vi "Configure Multi Eval Meas Limit SEM OBW.vi"(7 "Limit OBW (40e+6)":dbl=40000000.0 format="%^.3e", 8 "error in (no error)":errorcluster, 9 "Limit OBW Enabled (Value)":i32(ring)=2 items=["Off", "On", "Value"], 10 "Instance (1)":T1=1, 11 "VISA resource name":refnum<visa-resource-name>) -> (0 "error out":errorcluster, 3 "VISA resource name out":refnum<visa-resource-name>)   [LabVIEW 2020, in "Rohde&Schwarz CMWXP NR FR1 Measurement.lvlib"]
doc: "Defines an upper limit for the occupied bandwidth, for EN-DC measurements.\n\nAttributes:\nRSCMWXPNRFR1M_ATTR_MULTI_EVAL_MEAS_LIMIT_SEM_OBW_ENABLED\nRSCMWXPNRFR1M_ATTR_MULTI_EVAL_MEAS_LIMIT_SEM_OBW\n\nRemote-control command:\nCONFigure:NRSub:MEAS<i>:MEValuation:LIMit:SEMask:OBWLimit:ENDC"
uses:
  <instrlib>/Rohde&Schwarz CMWXP NR FR1 Measurement/Rohde&Schwarz CMWXP NR FR1 Measurement.lvlib
  <instrlib>/Rohde&Schwarz CMWXP NR FR1 Measurement/Private/_Instance.ctl
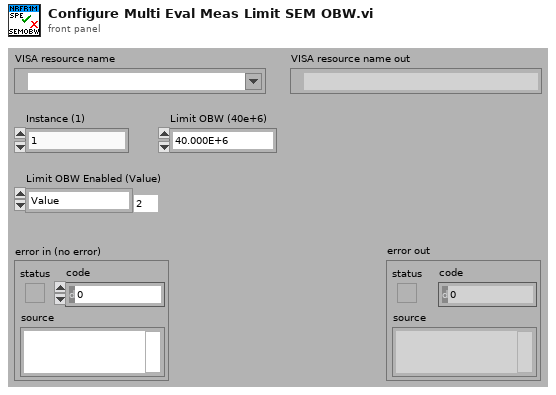
[diagram p1: front panel]
types:
  T1 = typedef "Rohde&Schwarz CMWXP NR FR1 Measurement.lvlib/_Instance.ctl" = i32
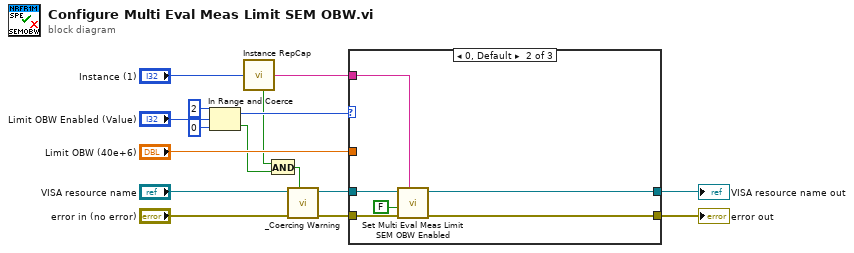
[diagram p0: block diagram]
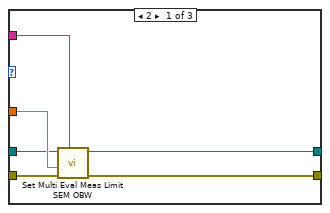
[diagram p2: hidden frame]
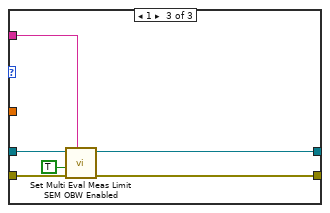
[diagram p3: hidden frame]
diagram:
  n1 = In Range and Coerce(upper limit=2, x="Limit OBW Enabled (Value)", lower limit=0) -> (coerced(x)=w12:i32, In Range?=w1:bool)
  n2 = call <instrlib>:"Instance RepCap.vi"("Instance In"="Instance (1)") -> ("In Range?"=w2:bool, "RepCap Identifier Out"=w8:string)  [unwired: 1 in]
  n3 = And(x=w2, y=w1) -> (x .and. y?=w3:bool)
  n4 = call <instrlib>:"_Coercing Warning.vi"("In Range?"=w3, "error in (no error)"="error in (no error)", "VISA resource name"="VISA resource name") -> ("error out"=w16:errorcluster, "VISA resource name out"=w15:refnum<visa-resource-name>)  [unwired: 7 in]
  n5 = case shown="0, Default" w12 {
    tunnel: [w22 w28 w34] -> w4
    tunnel: [w21 w27 w33] -> w5
    tunnel: "Limit OBW (40e+6)" -> [w20 _ _]
    tunnel: w16 -> [w19 w26 w32]
    tunnel: w15 -> [w18 w25 w31]
    tunnel: w8 -> [w17 w24 w30]
    frame 2 {
      n6 = call "Set Multi Eval Meas Limit SEM OBW"("Repeated Capabilities"=w17, "error in (no error)"=w19, "Multi Eval Meas Limit SEM OBW (0.0)"=w20, "instrument handle"=w18) -> ("error out"=w22:errorcluster, "instrument handle out"=w21:refnum<visa-resource-name>)  [unwired: 6 in]
    }
    frame 0, Default {
      n7 = call "Set Multi Eval Meas Limit SEM OBW Enabled"("Repeated Capabilities"=w24, "error in (no error)"=w26, "Multi Eval Meas Limit SEM OBW Enabled (OFF)"=FALSE ("Multi Eval Meas Limit OBW Enabled (OFF)"), "instrument handle"=w25) -> ("error out"=w28:errorcluster, "instrument handle out"=w27:refnum<visa-resource-name>)  [unwired: 6 in]
    }
    frame 1 {
      n8 = call "Set Multi Eval Meas Limit SEM OBW Enabled"("Repeated Capabilities"=w30, "error in (no error)"=w32, "Multi Eval Meas Limit SEM OBW Enabled (OFF)"=TRUE ("Multi Eval Meas Limit OBW Enabled (OFF)"), "instrument handle"=w31) -> ("error out"=w34:errorcluster, "instrument handle out"=w33:refnum<visa-resource-name>)  [unwired: 6 in]
    }
  }
  "error out" <- w4
  "VISA resource name out" <- w5
